vi "util_dialog_timeout_one_button.vi"(0 "Message text":string, 2 "Button text":string="OK", 3 "Timeout (s)":dbl=15.0 caption="Time Target (s)", 5 "Stopped":bool) -> ()   [LabVIEW 2016]
uses:
  user32.dll
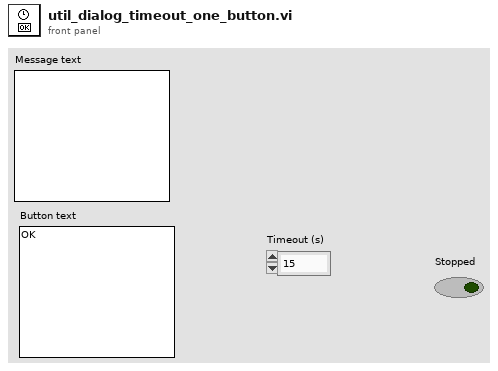
[diagram p1: front panel]
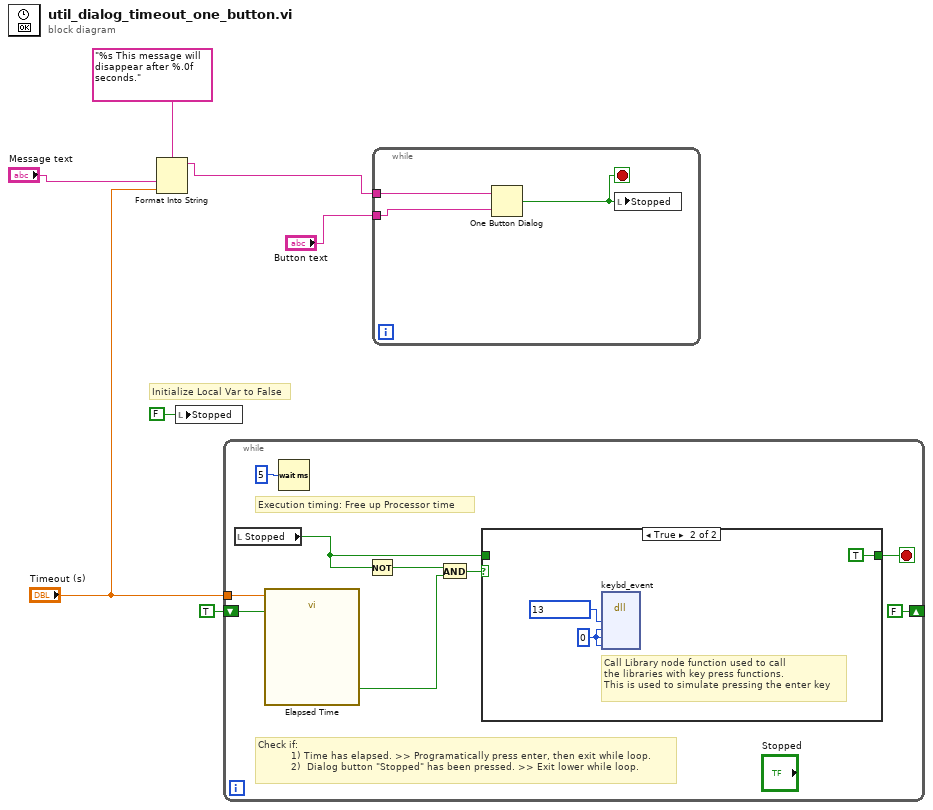
[diagram p0: block diagram]
diagram:
  # "Initialize Local Var to False"
  n1 = Format Into String(format string="%s This message will disappear after %.0f seconds.", "Message text", "Timeout (s)") -> (resulting string=w5:string)  [unwired: 2 in, 1 out]
  n2 = local write "Stopped"(FALSE ("Stopped")) -> ()
  n3 = while {
    tunnel: "Timeout (s)" -> [w11]
    shift-right: [FALSE] -> _
    shift-left: TRUE -> [w8]
    stop <- w16 stop-if-true
    # "Check if:\n           1) Time has elapsed. >> Programatically press enter, then exit while loop.\n           2)  Dialog button \"Stopped\" has been pressed. >> Exit lower while loop."
    # "Execution timing: Free up Processor time"
    n4 = local read "Stopped"() -> (w10:bool)
    n5 = call "Elapsed Time"("Time Target (s)"=w11, "Reset"=w8) -> ("Time has Elapsed"=w13:bool)  [unwired: 10 in, 7 out]
    n6 = Wait (ms)(milliseconds to wait=u32 5) -> ()  [unwired: 1 out]
    n7 = Not(x=w10) -> (.not. x?=w14:bool)
    n8 = And(x=w14, y=w13) -> (x .and. y?=w15:bool)
    n9 = case shown="True" w15 {
      tunnel: [w17 TRUE] -> w16
      tunnel: w10 -> [w17 _]
      frame False {
      }
      frame True {
        w19 = u8 0 ("bScan")
        # "Call Library node function used to call \nthe libraries with key press functions. \nThis is used to simulate pressing the enter key"
        n10 = dll-call lib="user32.dll" fn="keybd_event"("bVk"=u8 13 ("Virtual Key"), "bScan"=w19, "dwFlags"=w19, "dwExtraInfo"=w19) -> ()  [unwired: 8 in, 2 out]
      }
    }
  }
  n11 = while {
    tunnel: w5 -> [w22]
    tunnel: "Button text" -> [w21]
    stop <- w23 stop-if-true
    n12 = One Button Dialog(message=w22, button name ("OK")=w21) -> (true=w23:bool)
    n13 = local write "Stopped"(w23) -> ()
  }
